vi "Spectrometer_File_Naming.vi"(9 "Description":string, 10 "Sample MetaData Cluster":T1={"Sample Volume (uL)"=18.0, "Sample Mass (ug)"=0.45, "Sample Conc(mg/mL)"=0.025, "Sample Temperature (C)"=23.0, "Batch Num"=999.0, "Batch Name"="Test", "Solute"="Test", "Solvent"="Water", "Sample Description"="Test"}, 11 "Ring":u16(ring) items=["Spec.", "Mag.", "In Out Spec"]) -> (3 "Output Name":string)   [LabVIEW 2021]
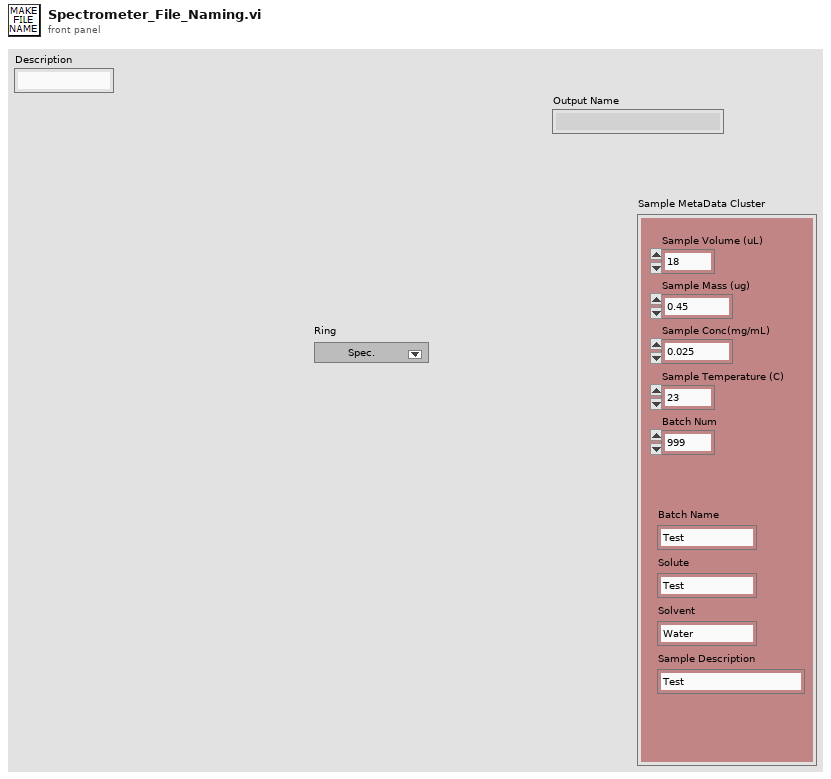
[diagram p1: front panel]
types:
  T1 = cluster{"Sample Volume (uL)":dbl, "Sample Mass (ug)":dbl, "Sample Conc(mg/mL)":dbl, "Sample Temperature (C)":dbl, "Batch Num":dbl, "Batch Name":string, "Solute":string, "Solvent":string, "Sample Description":string}
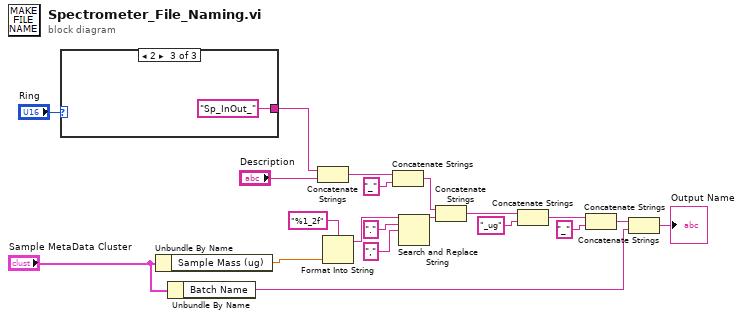
[diagram p0: block diagram]
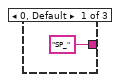
[diagram p2: hidden frame]
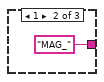
[diagram p3: hidden frame]
diagram:
  n1 = case shown="2" "Ring" {
    tunnel: ["SP_" ("string") "MAG_" ("string") "Sp_InOut_" ("string")] -> w4
    frame 0, Default {
    }
    frame 1 {
    }
    frame 2 {
    }
  }
  n2 = Unbundle By Name("Sample MetaData Cluster") -> ("Sample Mass (ug)"=w20:dbl)
  n3 = Unbundle By Name("Sample MetaData Cluster") -> ("Batch Name"=w11:string)
  n4 = Concatenate Strings(w4, "Description") -> (w3:string)
  n5 = Format Into String(format string="%1_2f", w20) -> (resulting string=w16:string)  [unwired: 2 in, 1 out]
  n6 = Concatenate Strings(w3, "_" ("string")) -> (w1:string)
  n7 = Search and Replace String(input string=w16, search string=".", replace string="," ("replace string (\"\")")) -> (result string=w13:string)  [unwired: 5 in, 3 out]
  n8 = Concatenate Strings(w1, w13) -> (w18:string)
  n9 = Concatenate Strings(w18, "_ug" ("string")) -> (w9:string)
  n10 = Concatenate Strings(w9, "_" ("string")) -> (w7:string)
  n11 = Concatenate Strings(w7, w11) -> (→"Output Name":string)
